vi "Get Pre Amp Gain.vi"(10 "gain":sgl, 11 "index":i32) -> (2 "gain out":sgl, 3 "function return":u32)   [LabVIEW 2018, in "AndorSDK.lvlib"]
doc: "EXPNETTYPE unsigned int WINAPI GetPreAmpGain(int index, float * gain);"
uses:
  AndorSDK.lvlib
  ATMCD32D.dll
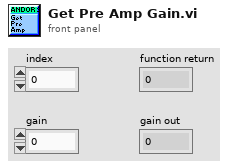
[diagram p1: front panel]
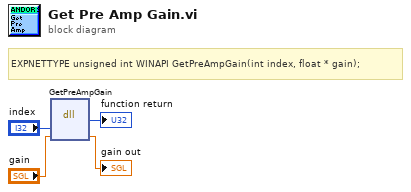
[diagram p0: block diagram]
diagram:
  # "EXPNETTYPE unsigned int WINAPI GetPreAmpGain(int index, float * gain);"
  n1 = dll-call lib="PTH2babs E\nPersönliches02 - Arbeit03-HiwijobsLabviewCodelibANDOR\tAndor SDK\nATMCD32D.*" fn="GetPreAmpGain"("index"="index", "gain"="gain") -> (→"function return":u32, "gain"=→"gain out":sgl)  [unwired: 4 in, 2 out]
